vi "combo_box_input.vi"(7 "callee":refnum<vi>, 8 "error in (no error)":errorcluster, 11 "configuration":T2={"dialog_text"="", "boolean_text_1"="", "boolean_text_2"="", "boolean_text_3"="", "inner_color"=16711680, "outer_color"=6618880, "wait_s"=nan, "error_status"=FALSE, "error_source"="", "error_details"="", "string []"=[], "custom_entry"=FALSE}) -> (0 "error out":errorcluster, 2 "value":string, 3 "dialog_selection":T1)   [LabVIEW 2015, in "lv-dialog-interfaces.lvlib"]
uses:
  lv-dialog-interfaces.lvlib
  lv-dialog/api/v1/public/_controls/configuration.ctl
  lv-dialog/api/v1/public/_controls/dialog_selection.ctl
  _controls/dialog_type.ctl
  _controls/hmi_references.ctl
  <vilib>/event_ctls.llb/eventvkey.ctl
  lv-dialog/api/v1/v1.lvlib
panel:
  out "dialog":string
  in  "combo_box":string(combo)
  in  "button_1":bool
  in  "button_2":bool
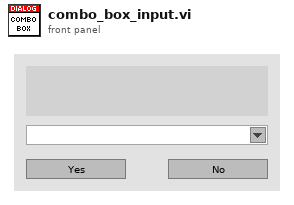
[diagram p1: front panel]
types:
  T1 = typedef "lv-dialog.lvlib/v1.lvlib/dialog_selection.ctl" = enum16{"null", "panel_closed", "button_1", "button_2", "button_3", "cancelled"}
  T2 = typedef "lv-dialog.lvlib/v1.lvlib/configuration.ctl" = cluster{"dialog_text":string, "boolean_text_1":string, "boolean_text_2":string, "boolean_text_3":string, "inner_color":u32, "outer_color":u32, "wait_s":dbl, "error_status":bool, "error_source":string, "error_details":string, "string []":string[], "custom_entry":bool}
  T3 = typedef "lv-dialog-interfaces.lvlib/dialog_type.ctl" = enum16{"null", "one_button", "two_button", "three_button", "confirmation", "busy_wait", "error", "busy_wait_embed", "combo_box", "data_entry_string", "data_entry_numeric"}
  T4 = typedef "lv-dialog-interfaces.lvlib/hmi_references.ctl" = cluster{"vi_reference":refnum<vi>, "caller":refnum<vi>, "dialog":refnum<vi>, "button_1":refnum<vi>, "button_2":refnum<vi>, "button_3":refnum<vi>, "busy":refnum<vi>, "error_glyph":refnum<vi>, "error_source":refnum<vi>, "error_text":refnum<vi>, "combo_box":refnum<vi>}
  T5 = typedef "eventvkey.ctl" = enum16{"ASCII", "Enter", "Return", "Shift", "Ctrl", "Alt", "Cmd", "Opt", "Caps", "NumLock", "Clear", "Break", "Up", "Down", "Left", "Right", "Insert", "Delete", "Home", "End", "PageUp", "PageDown", "Escape", "Help", "Pause", "ScrollLock", "F1", "F2", "F3", "F4", "F5", "F6", "F7", "F8", "F9", "F10", "F11", "F12", "F13", "F14", "F15", "F16", "F17", "F18", "F19", "F20", "F21", "F22", "F23", "F24", "Play", "VolumeUp", "VolumeDown", "Mute", "Two Byte Char"}
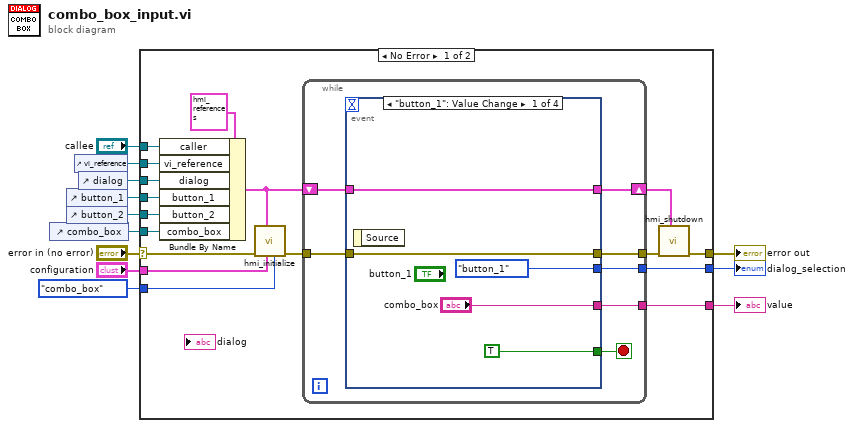
[diagram p0: block diagram]
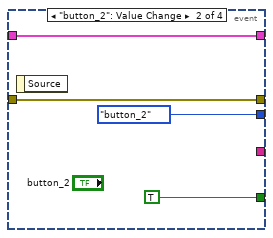
[diagram p2: hidden frame]
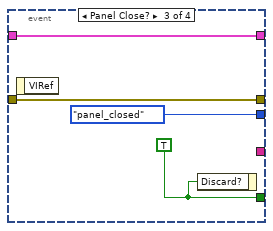
[diagram p3: hidden frame]
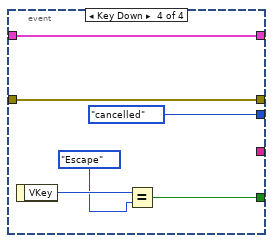
[diagram p4: hidden frame]
diagram:
  n1 = control-ref of="combo_box"() -> (w2:refnum<vi>)
  n2 = control-ref of="button_1"() -> (w4:refnum<vi>)
  n3 = control-ref of="button_2"() -> (w3:refnum<vi>)
  n4 = control-ref of="vi_reference"() -> (w6:refnum<vi>)
  n5 = control-ref of="dialog"() -> (w5:refnum<vi>)
  n6 = case shown="No Error" "error in (no error)" {
    selector: "error in (no error)" -> [w29 w56]
    tunnel: "configuration" -> [w28 _]
    tunnel: dialog_type."combo_box" ("dialog_type") -> [w27 _]
    tunnel: [w25 _] -> w9
    tunnel: "callee" -> [w24 _]
    tunnel: [w22 w56] -> w7
    tunnel: w6 -> [w19 _]
    tunnel: w5 -> [w14 _]
    tunnel: w4 -> [w15 _]
    tunnel: w3 -> [w16 _]
    tunnel: w2 -> [w17 _]
    tunnel: [w13 _] -> w1
    frame No Error {
      n7 = Bundle By Name(cluster=T4 {"vi_reference"=refnum, "caller"=refnum, "dialog"=refnum, "button_1"=refnum, "button_2"=refnum, "button_3"=refnum, "busy"=refnum, "error_glyph"=refnum, "error_source"=refnum, "error_text"=refnum, "combo_box"=refnum}, "caller"=w24, "vi_reference"=w19, "dialog"=w14, "button_1"=w15, "button_2"=w16, "combo_box"=w17) -> (w21:T4)
      n8 = call "hmi_initialize.vi"("dialog_type"=w27, "configuration"=w28, "references"=w21, "error in (no error)"=w29) -> ("error out"=w26:errorcluster)  [unwired: 7 in]
      n9 = while {
        tunnel: [w34] -> w25
        shift-right: [w32] -> w20
        shift-left: w21 -> [w33]
        tunnel: w26 -> [w36]
        tunnel: [w35] -> w23
        tunnel: [w30] -> w13
        stop <- w31 stop-if-true
        n10 = event shown="[0] \"button_1\": Value Change" {
          selector: _ -> [_ _ _ _]
          dyn-events: _ -> [_ _ _ _]
          timeout: _ -> [_ _ _ _]
          tunnel: w36 -> [w41 w45 w49 w55]
          tunnel: [w41 w45 w49 w55] -> w35
          tunnel: [dialog_selection."button_1" ("dialog_selection") dialog_selection."button_2" ("dialog_selection") dialog_selection."panel_closed" ("dialog_selection") dialog_selection."cancelled" ("dialog_selection")] -> w34
          tunnel: w33 -> [w39 w43 w47 w53]
          tunnel: [w39 w43 w47 w53] -> w32
          tunnel: [TRUE ("Discard?") TRUE ("Discard?") w46 w52] -> w31
          tunnel: ["combo_box" _ _ _] -> w30
          event "button_1": Value Change {
            n11 = event-data() -> ()  [unwired: 1 in, 1 out]
          }
          event "button_2": Value Change {
            n12 = event-data() -> ()  [unwired: 1 in, 1 out]
          }
          event Panel Close? {
            w46 = TRUE ("Discard?")
            n13 = event-data() -> ()  [unwired: 1 in, 1 out]
            n14 = event-data("Discard?"=w46) -> ()  [unwired: 1 in, 1 out]
          }
          event Key Down {
            n15 = event-data() -> ("VKey"=w51:T5)  [unwired: 1 in]
            n16 = Equal?(x=w51, y=eventvkey."Escape" ("VKey")) -> (x = y?=w52:bool)
          }
        }
      }
      n17 = call "hmi_shutdown.vi"("references"=w20, "error in (no error)"=w23) -> ("error out"=w22:errorcluster)  [unwired: 9 in]
    }
    frame Error {
    }
  }
  "error out" <- w7
  "dialog_selection" <- w9
  "value" <- w1
